vi "onlycam.vi"() -> ()   [LabVIEW 2014]
panel:
  in  "AOI Width":i32=2560
  in  "AOI Height":i32=2160
  out "Status":i32
  out "error":errorcluster
  in  "PreAmp Gain Control":string(combo)
  in  "ExposureTime":dbl=0.1
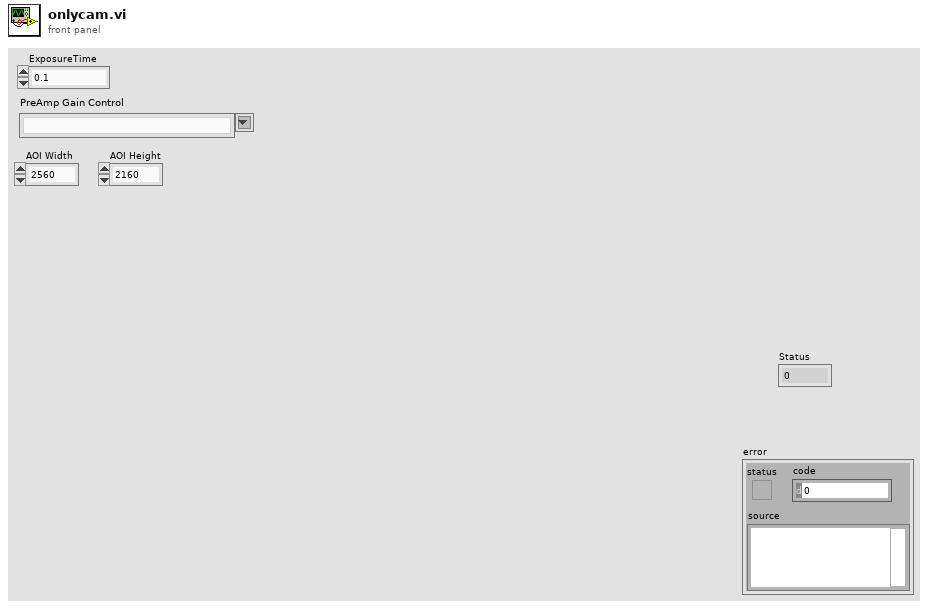
[diagram p1: front panel]
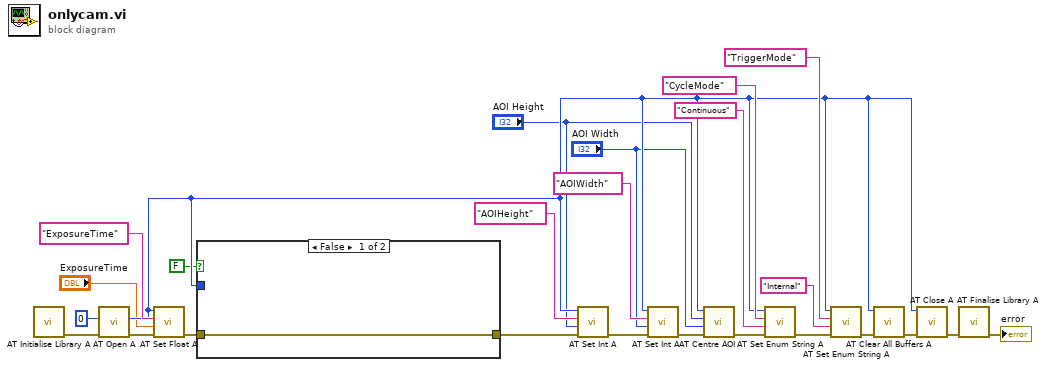
[diagram p0: block diagram]
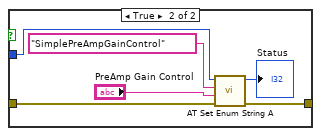
[diagram p2: hidden frame]
diagram:
  n1 = call <userlib>:"AT Initialise Library A.vi"() -> ("error out"=w24:errorcluster)  [unwired: 10 in, 1 out]
  n2 = call <userlib>:"AT Open A.vi"("error in (no error)"=w24, "CameraIndex"=0) -> ("error out"=w17:errorcluster, "Handle"=w5:i32)  [unwired: 7 in, 1 out]
  n3 = call <userlib>:"AT Set Float A.vi"("error in (no error)"=w17, "Value"="ExposureTime", "Feature"="ExposureTime" ("ExposureTime"), "Hndl"=w5) -> ("error out"=w23:errorcluster)  [unwired: 6 in, 1 out]
  n4 = case shown="False" FALSE {
    tunnel: w23 -> [w26 w32]
    tunnel: [w26 w31] -> w21
    tunnel: w5 -> [_ w28]
    frame False {
    }
    frame True {
      n5 = call <userlib>:"AT Set Enum String A.vi"("error in (no error)"=w32, "String"="PreAmp Gain Control", "Feature"="SimplePreAmpGainControl" ("Enum feature"), "Handle"=w28) -> ("error out"=w31:errorcluster, "Status"=→"Status":i32)  [unwired: 6 in]
    }
  }
  n6 = call <userlib>:"AT Set Int A.vi"("error in (no error)"=w21, "Value"="AOI Height", "Feature"="AOIHeight" ("Integer feature"), "Handle"=w5) -> ("error out"=w20:errorcluster)  [unwired: 6 in, 1 out]
  n7 = call <userlib>:"AT Set Int A.vi"("error in (no error)"=w20, "Value"="AOI Width", "Feature"="AOIWidth" ("Integer feature 2"), "Handle"=w5) -> ("error out"=w16:errorcluster)  [unwired: 6 in, 1 out]
  n8 = call <userlib>:"AT Centre AOI.vi"("error in (no error)"=w16, "AOI Width"="AOI Width", "AOI Height"="AOI Height", "Handle"=w5) -> ("error out"=w10:errorcluster)  [unwired: 7 in]
  n9 = call <userlib>:"AT Set Enum String A.vi"("error in (no error)"=w10, "String"="Continuous", "Feature"="CycleMode" ("Enum feature"), "Handle"=w5) -> ("error out"=w14:errorcluster)  [unwired: 6 in, 1 out]
  n10 = call <userlib>:"AT Set Enum String A.vi"("error in (no error)"=w14, "String"="Internal", "Feature"="TriggerMode" ("Enum feature"), "Handle"=w5) -> ("error out"=w7:errorcluster)  [unwired: 6 in, 1 out]
  n11 = call <userlib>:"AT Clear All Buffers A.vi"("error in (no error)"=w7, "Handle"=w5) -> ("error out"=w8:errorcluster)  [unwired: 8 in, 1 out]
  n12 = call <userlib>:"AT Close A.vi"("error in (no error)"=w8, "Handle"=w5) -> ("error out"=w9:errorcluster)  [unwired: 8 in, 1 out]
  n13 = call <userlib>:"AT Finalise Library A.vi"("error in (no error)"=w9) -> ("error out"=→"error":errorcluster)  [unwired: 9 in, 1 out]
